vi "read named variant G.vi"() -> ()   [LabVIEW 2014]
uses:
  <vilib>/Utility/config.llb/NI_LVConfig.lvlib
panel:
  out "data":T1 {"Contours"."Type" items=["No Selection", "Point", "Line", "Rectangle", "Oval", "Polygon", "Freehand Region", "Annulus", "Unused2", "Unused3", "Broken Line", "Freehand Line", "Rotated Rectangle"]}
  out "Section Formatted Cluster":variant
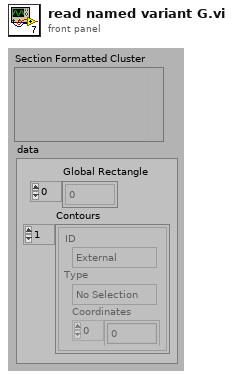
[diagram p1: front panel]
types:
  T1 = typedef "ROI Descriptor" = cluster{"Global Rectangle":i32[], "Contours":cluster{"ID":enum32{"External", "Internal"}, "Type":u32, "Coordinates":i32[]}[]}
  T2 = typedef "NI_LVConfig.lvlib/Config Data RefNum.ctl" = refnum<k1>
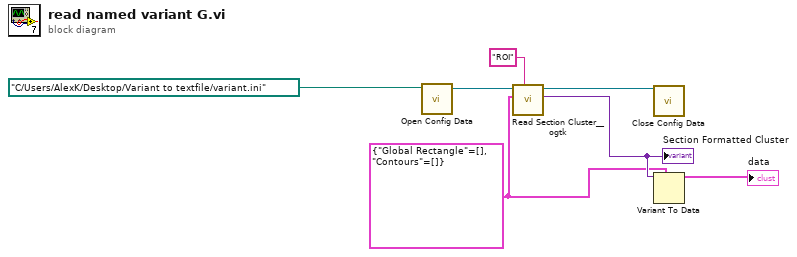
[diagram p0: block diagram]
diagram:
  w2 = T1 {"Global Rectangle"=[], "Contours"=[]} ("ROI Descriptor")
  n1 = call <vilib>:"Open Config Data.vi"("configuration file path"=path "C:/Users/AlexK/Desktop/Variant to textfile/variant.ini" ("file (use dialog)")) -> ("refnum"=w6:T2)  [unwired: 8 in, 2 out]
  n2 = call <userlib>:"Read Section Cluster__ogtk.vi"("section (optional)"="ROI", "Section Formatted Cluster Type"=w2, "refnum"=w6) -> ("Section Formatted Cluster"=w3:variant, "dup refnum"=w4:T2)  [unwired: 4 in, 3 out]
  "Section Formatted Cluster" <- w3
  n3 = call <vilib>:"Close Config Data.vi"("refnum"=w4) -> ()  [unwired: 9 in, 2 out]
  n4 = Variant To Data(type=w2, Variant=w3) -> (data=→"data":T1)  [unwired: 1 in, 1 out]
